vi "ChSetting - 副本.vi"(10 "dsc地址":string, 11 "AcquireData":waveform(dbl)[](array[waveform])) -> (1 "DexASData":T1, 2 "DevChSampData":cluster{"通道编号":string, "Data":dbl}[](array[cluster]), 3 "DevChSampleData":T2)   [LabVIEW 2014]
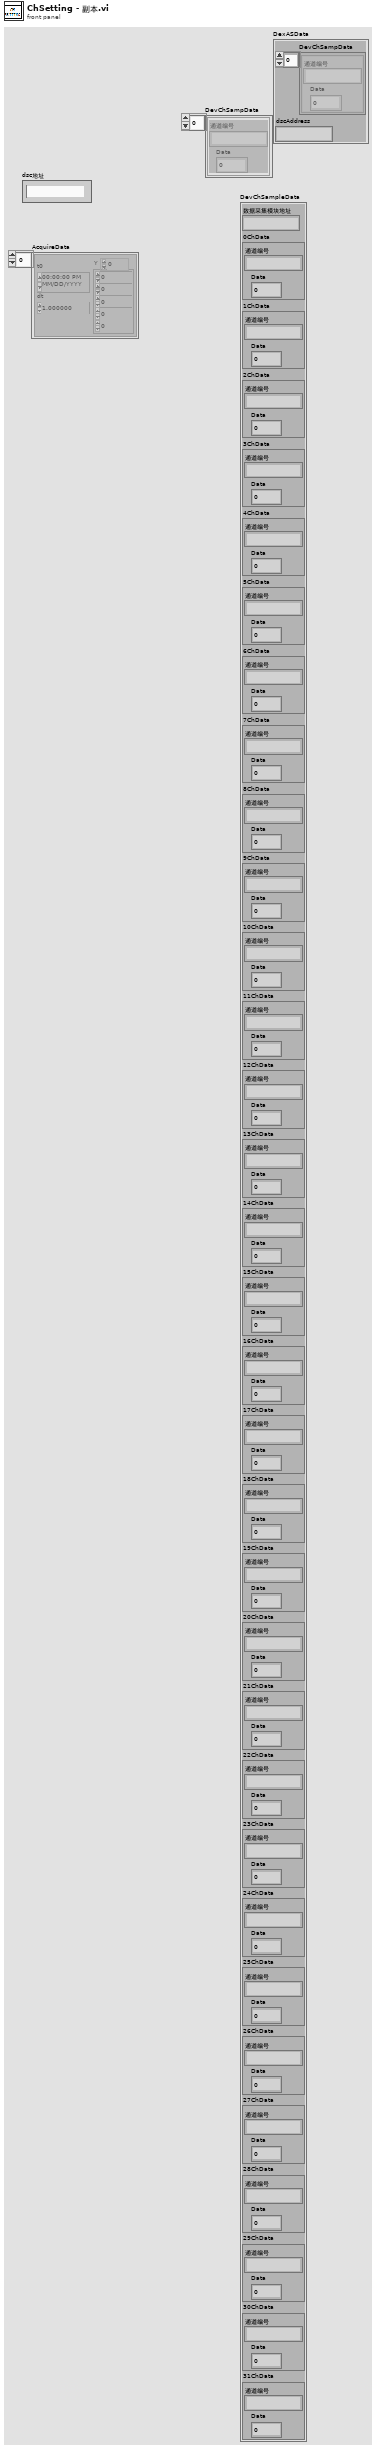
[diagram p1: front panel]
types:
  T1 = cluster{"DevChSampData":cluster{"通道编号":string, "Data":dbl}[], "dscAddress":string}
  T2 = cluster{"数据采集模块地址":string, "0ChData":cluster{"通道编号":string, "Data":dbl}, "1ChData":cluster{"通道编号":string, "Data":dbl}, "2ChData":cluster{"通道编号":string, "Data":dbl}, "3ChData":cluster{"通道编号":string, "Data":dbl}, "4ChData":cluster{"通道编号":string, "Data":dbl}, "5ChData":cluster{"通道编号":string, "Data":dbl}, "6ChData":cluster{"通道编号":string, "Data":dbl}, "7ChData":cluster{"通道编号":string, "Data":dbl}, "8ChData":cluster{"通道编号":string, "Data":dbl}, "9ChData":cluster{"通道编号":string, "Data":dbl}, "10ChData":cluster{"通道编号":string, "Data":dbl}, "11ChData":cluster{"通道编号":string, "Data":dbl}, "12ChData":cluster{"通道编号":string, "Data":dbl}, "13ChData":cluster{"通道编号":string, "Data":dbl}, "14ChData":cluster{"通道编号":string, "Data":dbl}, "15ChData":cluster{"通道编号":string, "Data":dbl}, "16ChData":cluster{"通道编号":string, "Data":dbl}, "17ChData":cluster{"通道编号":string, "Data":dbl}, "18ChData":cluster{"通道编号":string, "Data":dbl}, "19ChData":cluster{"通道编号":string, "Data":dbl}, "20ChData":cluster{"通道编号":string, "Data":dbl}, "21ChData":cluster{"通道编号":string, "Data":dbl}, "22ChData":cluster{"通道编号":string, "Data":dbl}, "23ChData":cluster{"通道编号":string, "Data":dbl}, "24ChData":cluster{"通道编号":string, "Data":dbl}, "25ChData":cluster{"通道编号":string, "Data":dbl}, "26ChData":cluster{"通道编号":string, "Data":dbl}, "27ChData":cluster{"通道编号":string, "Data":dbl}, "28ChData":cluster{"通道编号":string, "Data":dbl}, "29ChData":cluster{"通道编号":string, "Data":dbl}, "30ChData":cluster{"通道编号":string, "Data":dbl}, "31ChData":cluster{"通道编号":string, "Data":dbl}}
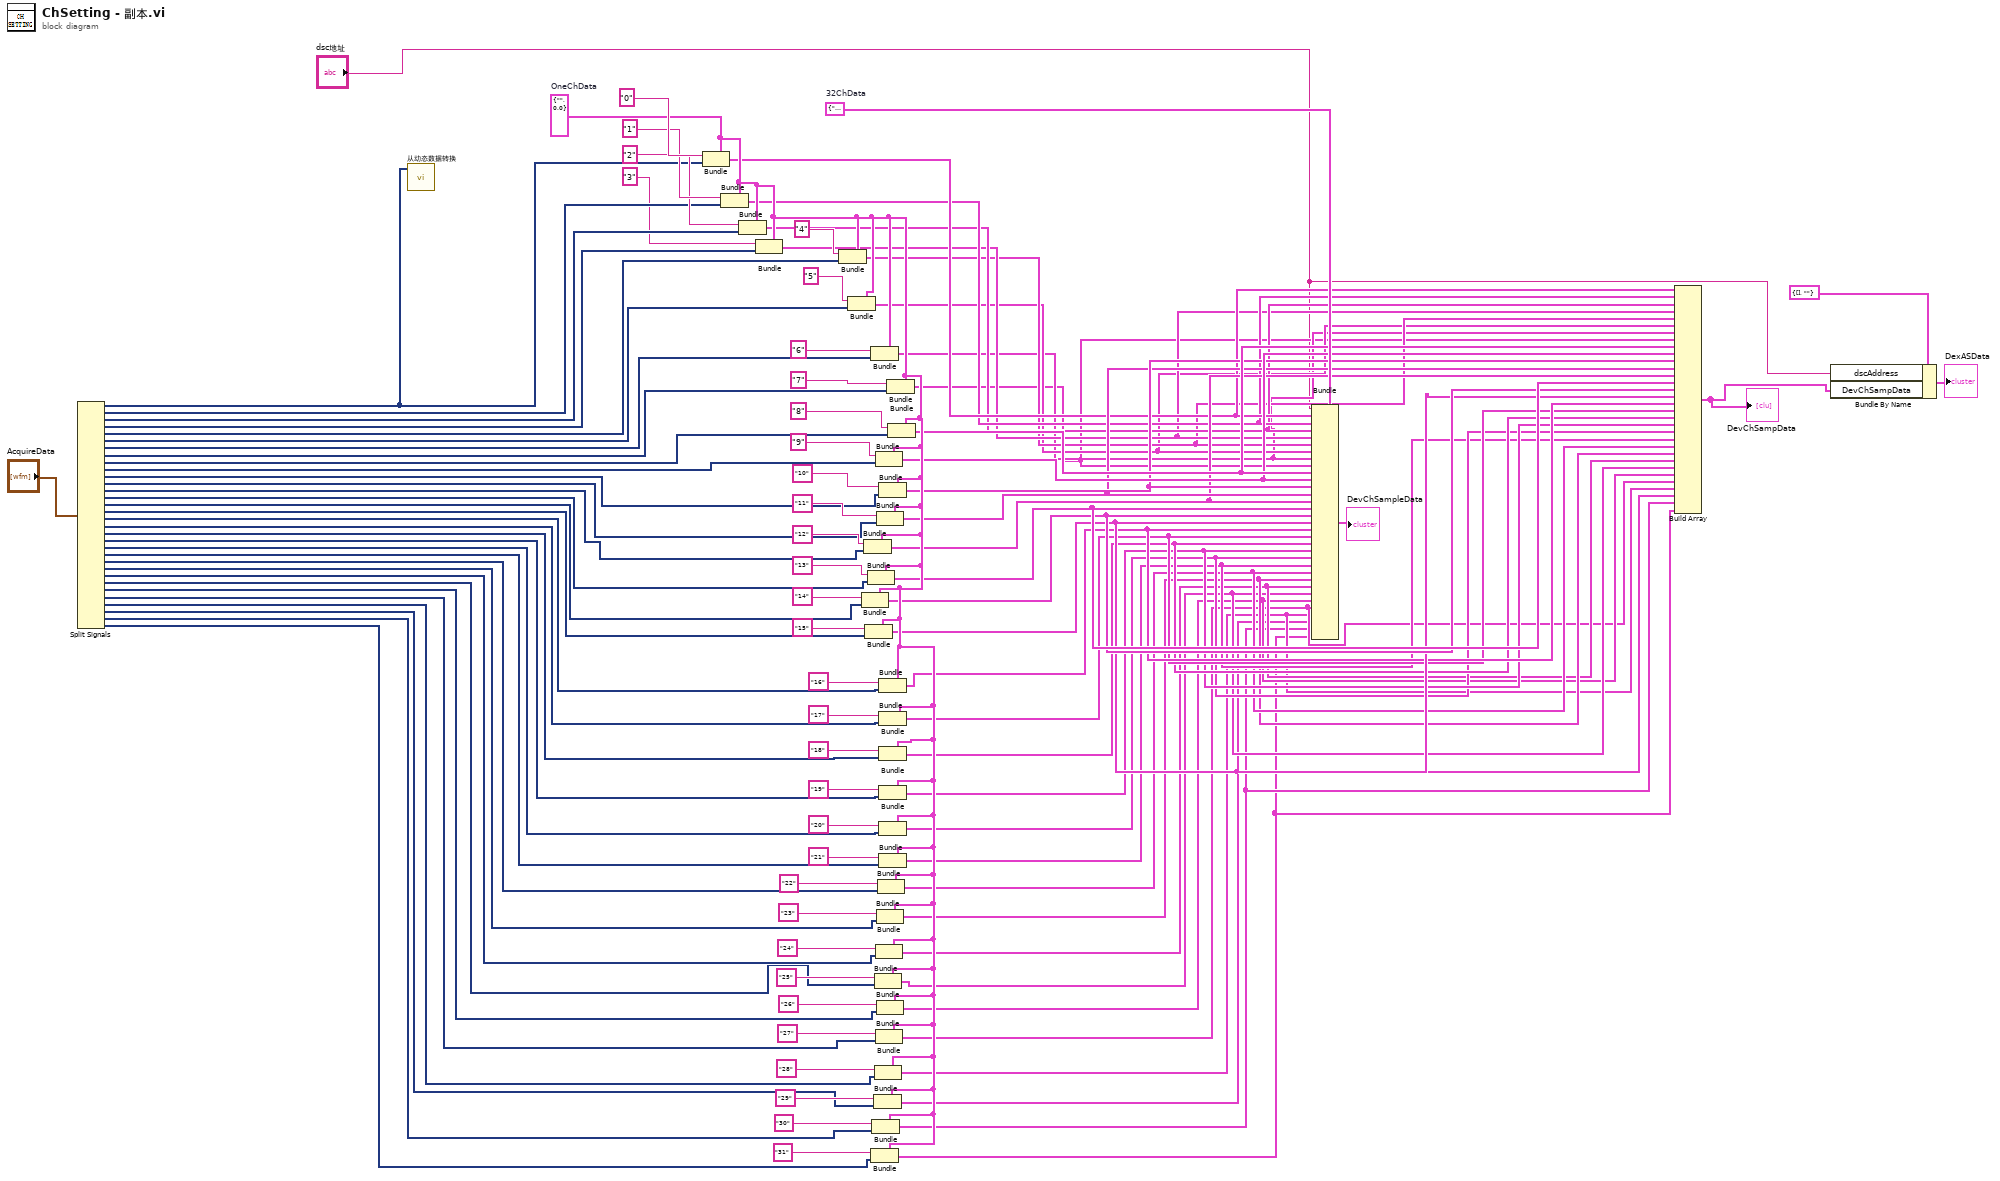
[diagram p0: block diagram]
diagram:
  w85 = T2 {"数据采集模块地址"="", "0ChData"={"通道编号"="", "Data"=0.0}, "1ChData"={"通道编号"="", "Data"=0.0}, "2ChData"={"通道编号"="", "Data"=0.0}, "3ChData"={"通道编号"="", "Data"=0.0}, "4ChData"={"通道编号"="", "Data"=0.0}, "5ChData"={"通道编号"="", "Data"=0.0}, "6ChData"={"通道编号"="", "Data"=0.0}, "7ChData"={"通道编号"="", "Data"=0.0}, "8ChData"={"通道编号"="", "Data"=0.0}, "9ChData"={"通道编号"="", "Data"=0.0}, "10ChData"={"通道编号"="", "Data"=0.0}, "11ChData"={"通道编号"="", "Data"=0.0}, "12ChData"={"通道编号"="", "Data"=0.0}, "13ChData"={"通道编号"="", "Data"=0.0}, "14ChData"={"通道编号"="", "Data"=0.0}, "15ChData"={"通道编号"="", "Data"=0.0}, "16ChData"={"通道编号"="", "Data"=0.0}, "17ChData"={"通道编号"="", "Data"=0.0}, "18ChData"={"通道编号"="", "Data"=0.0}, "19ChData"={"通道编号"="", "Data"=0.0}, "20ChData"={"通道编号"="", "Data"=0.0}, "21ChData"={"通道编号"="", "Data"=0.0}, "22ChData"={"通道编号"="", "Data"=0.0}, "23ChData"={"通道编号"="", "Data"=0.0}, "24ChData"={"通道编号"="", "Data"=0.0}, "25ChData"={"通道编号"="", "Data"=0.0}, "26ChData"={"通道编号"="", "Data"=0.0}, "27ChData"={"通道编号"="", "Data"=0.0}, "28ChData"={"通道编号"="", "Data"=0.0}, "29ChData"={"通道编号"="", "Data"=0.0}, "30ChData"={"通道编号"="", "Data"=0.0}, "31ChData"={"通道编号"="", "Data"=0.0}}  # 32ChData
  w48 = cluster{"通道编号":string, "Data":dbl} {"通道编号"="", "Data"=0.0}  # OneChData
  n1 = Split Signals("AcquireData") -> (w1:dynamicdata, w100:dynamicdata, w99:dynamicdata, w97:dynamicdata, w95:dynamicdata, w90:dynamicdata, w89:dynamicdata, w88:dynamicdata, w79:dynamicdata, w78:dynamicdata, w77:dynamicdata, w76:dynamicdata, w75:dynamicdata, w74:dynamicdata, w73:dynamicdata, w72:dynamicdata, w65:dynamicdata, w64:dynamicdata, w63:dynamicdata, w62:dynamicdata, w61:dynamicdata, w60:dynamicdata, w49:dynamicdata, w47:dynamicdata, w46:dynamicdata, w45:dynamicdata, w44:dynamicdata, w43:dynamicdata, w42:dynamicdata, w41:dynamicdata, w40:dynamicdata, w39:dynamicdata)  [unwired: 32 in]
  n2 = call "从动态数据转换"("Dynamic Data Type"=w1) -> ()  [unwired: 3 in, 1 out]
  n3 = Bundle(cluster=w48, "通道编号"="0", "Data"=w1) -> (w13:cluster{"通道编号":string, "Data":dbl})
  n4 = Bundle(cluster=w48, "通道编号"="1", "Data"=w100) -> (w12:cluster{"通道编号":string, "Data":dbl})
  n5 = Bundle(cluster=w48, "通道编号"="2", "Data"=w99) -> (w11:cluster{"通道编号":string, "Data":dbl})
  n6 = Bundle(cluster=w48, "通道编号"="3", "Data"=w97) -> (w10:cluster{"通道编号":string, "Data":dbl})
  n7 = Bundle(cluster=w48, "通道编号"="4", "Data"=w95) -> (w9:cluster{"通道编号":string, "Data":dbl})
  n8 = Bundle(cluster=w48, "通道编号"="5", "Data"=w90) -> (w8:cluster{"通道编号":string, "Data":dbl})
  n9 = Bundle(cluster=w48, "通道编号"="14", "Data"=w73) -> (w31:cluster{"通道编号":string, "Data":dbl})
  n10 = Bundle(cluster=w48, "通道编号"="12", "Data"=w75) -> (w33:cluster{"通道编号":string, "Data":dbl})
  n11 = Bundle(cluster=w48, "通道编号"="15", "Data"=w72) -> (w30:cluster{"通道编号":string, "Data":dbl})
  n12 = Bundle(cluster=w48, "通道编号"="13", "Data"=w74) -> (w32:cluster{"通道编号":string, "Data":dbl})
  n13 = Bundle(cluster=w48, "通道编号"="6", "Data"=w89) -> (w7:cluster{"通道编号":string, "Data":dbl})
  n14 = Bundle(cluster=w48, "通道编号"="31", "Data"=w39) -> (w14:cluster{"通道编号":string, "Data":dbl})
  n15 = Bundle(cluster=w48, "通道编号"="30", "Data"=w40) -> (w15:cluster{"通道编号":string, "Data":dbl})
  n16 = Bundle(cluster=w48, "通道编号"="29", "Data"=w41) -> (w16:cluster{"通道编号":string, "Data":dbl})
  n17 = Bundle(cluster=w48, "通道编号"="25", "Data"=w45) -> (w20:cluster{"通道编号":string, "Data":dbl})
  n18 = Bundle(cluster=w48, "通道编号"="28", "Data"=w42) -> (w17:cluster{"通道编号":string, "Data":dbl})
  n19 = Bundle(cluster=w48, "通道编号"="9", "Data"=w78) -> (w36:cluster{"通道编号":string, "Data":dbl})
  n20 = Bundle(cluster=w48, "通道编号"="24", "Data"=w46) -> (w21:cluster{"通道编号":string, "Data":dbl})
  n21 = Bundle(cluster=w48, "通道编号"="27", "Data"=w43) -> (w18:cluster{"通道编号":string, "Data":dbl})
  n22 = Bundle(cluster=w48, "通道编号"="11", "Data"=w76) -> (w34:cluster{"通道编号":string, "Data":dbl})
  n23 = Bundle(cluster=w48, "通道编号"="23", "Data"=w47) -> (w22:cluster{"通道编号":string, "Data":dbl})
  n24 = Bundle(cluster=w48, "通道编号"="26", "Data"=w44) -> (w19:cluster{"通道编号":string, "Data":dbl})
  n25 = Bundle(cluster=w48, "通道编号"="22", "Data"=w49) -> (w23:cluster{"通道编号":string, "Data":dbl})
  n26 = Bundle(cluster=w48, "通道编号"="10", "Data"=w77) -> (w35:cluster{"通道编号":string, "Data":dbl})
  n27 = Bundle(cluster=w48, "通道编号"="16", "Data"=w65) -> (w29:cluster{"通道编号":string, "Data":dbl})
  n28 = Bundle(cluster=w48, "通道编号"="17", "Data"=w64) -> (w28:cluster{"通道编号":string, "Data":dbl})
  n29 = Bundle(cluster=w48, "通道编号"="18", "Data"=w63) -> (w27:cluster{"通道编号":string, "Data":dbl})
  n30 = Bundle(cluster=w48, "通道编号"="19", "Data"=w62) -> (w26:cluster{"通道编号":string, "Data":dbl})
  n31 = Bundle(cluster=w48, "通道编号"="20", "Data"=w61) -> (w25:cluster{"通道编号":string, "Data":dbl})
  n32 = Bundle(cluster=w48, "通道编号"="21", "Data"=w60) -> (w24:cluster{"通道编号":string, "Data":dbl})
  n33 = Bundle(cluster=w48, "通道编号"="7", "Data"=w88) -> (w6:cluster{"通道编号":string, "Data":dbl})
  n34 = Bundle(cluster=w48, "通道编号"="8", "Data"=w79) -> (w37:cluster{"通道编号":string, "Data":dbl})
  n35 = Bundle(cluster=w85, "数据采集模块地址"="dsc地址", "0ChData"=w13, "1ChData"=w12, "2ChData"=w11, "3ChData"=w10, "4ChData"=w9, "5ChData"=w8, "6ChData"=w7, "7ChData"=w6, "8ChData"=w37, "9ChData"=w36, "10ChData"=w35, "11ChData"=w34, "12ChData"=w33, "13ChData"=w32, "14ChData"=w31, "15ChData"=w30, "16ChData"=w29, "17ChData"=w28, "18ChData"=w27, "19ChData"=w26, "20ChData"=w25, "21ChData"=w24, "22ChData"=w23, "23ChData"=w22, "24ChData"=w21, "25ChData"=w20, "26ChData"=w19, "27ChData"=w18, "28ChData"=w17, "29ChData"=w16, "30ChData"=w15, "31ChData"=w14) -> (→"DevChSampleData":T2)
  n36 = Build Array(w13, w12, w11, w10, w9, w8, w7, w6, w37, w36, w35, w34, w33, w32, w31, w30, w29, w28, w27, w26, w25, w24, w23, w22, w21, w20, w19, w18, w17, w16, w15, w14) -> (w3:cluster{"通道编号":string, "Data":dbl}[])
  "DevChSampData" <- w3
  n37 = Bundle By Name(cluster=T1 {"DevChSampData"=[], "dscAddress"=""} ("dscAsampledata"), "dscAddress"="dsc地址", "DevChSampData"=w3) -> (→"DexASData":T1)
